vi "PicoScope2000aExampleRapidBlock.vi"() -> ()   [LabVIEW 2009]
panel:
  in  "Channel A Settings":T1 {"Range" items=["20 mV", "50 mV", "100 mV", "200 mV", "500 mV", "1 V", "2 V", "5 V", "10 V", "20 V"]; "Coupling" items=["AC", "DC"]}
  out "Properties Panel":T2 {"Max Total Capture Time Available (sec)" format="%.3p"; "Sample Frequency" format="%.3p"; "Sample Internal" format="%.3p"; "Max Samples Available" format="%.3p"; "Total Capture Time (sec)" format="%.3p"}
  in  "Down Sample Ratio":u32 min=1 step=1
  in  "Down-Sample Mode":i32(ring) items=["None", "Aggregate", "Decimate", "Average"]
  in  "Trigger Settings":T3 {"Trigger Direction" items=["Rising", "Falling"]}
  in  "Rapid Block Acquisition Settings":T4
  out "Capture Complete":bool
  in  "Run":bool
  out "Channel A":T5(graph)
  in  "Capture Index":u32
  in  "stop":bool
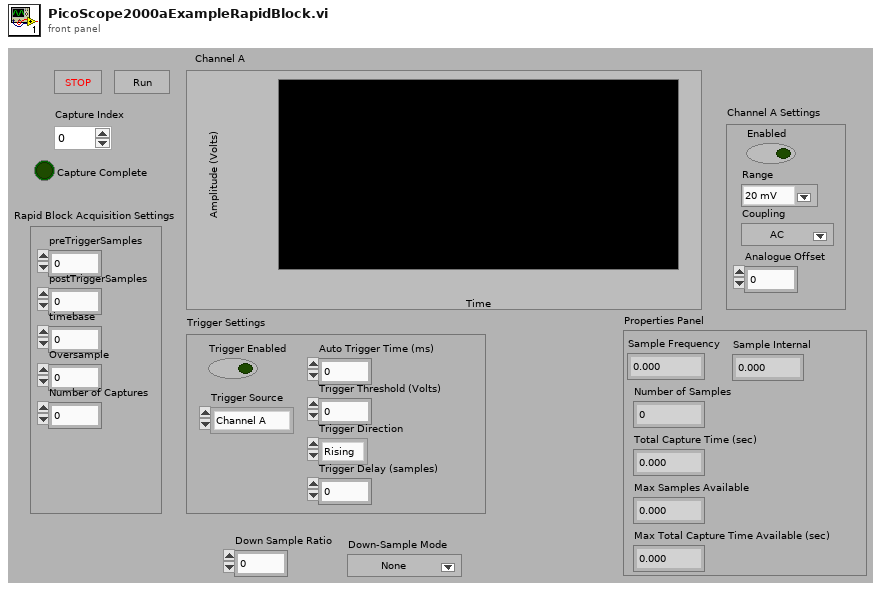
[diagram p1: front panel]
types:
  T1 = cluster{"Enabled":bool, "Coupling":i16, "Range":u16, "Analogue Offset":sgl}
  T2 = cluster{"Sample Frequency":sgl, "Sample Internal":sgl, "Max Samples Available":i32, "Number of Samples":u32, "Total Capture Time (sec) ":sgl, "Max Total Capture Time Available (sec)":sgl}
  T3 = cluster{"Trigger Enabled":bool, "Trigger Source":enum16{"Channel A", "Channel B", "Channel C", "Channel D", "Ext."}, "Trigger Threshold (Volts)":dbl, "Trigger Direction":u16, "Trigger Delay (samples)":u32, "Auto Trigger Time (ms)":i16}
  T4 = cluster{"preTriggerSamples":u32, "postTriggerSamples":u32, "timebase":u32, "Oversample":i16, "Number of Captures":u32}
  T5 = cluster{i32, "Sample Internal":sgl, "Data (Volts)":dbl[]}
  T6 = cluster{"Driver Version":string, "USB Version":string, "Hardware":string, "Variant":string, "Batch and Serial":string, "Cal Date":string, "Kernel Version":string, "Digital HW Version":string, "Analogue HW Version":string, "Firmware 1":string, "Firmware 2":string, "MSO":bool, "Number of Channels":i16}
  T7 = cluster{"preTriggerSamples":u32, "postTriggerSamples":u32, "timebase":u32, "Down-Sample Mode":i32, "Down Sample Ratio":u32, i16}
  T8 = cluster{i32, "Sample Internal":sgl, "Data":dbl[]}
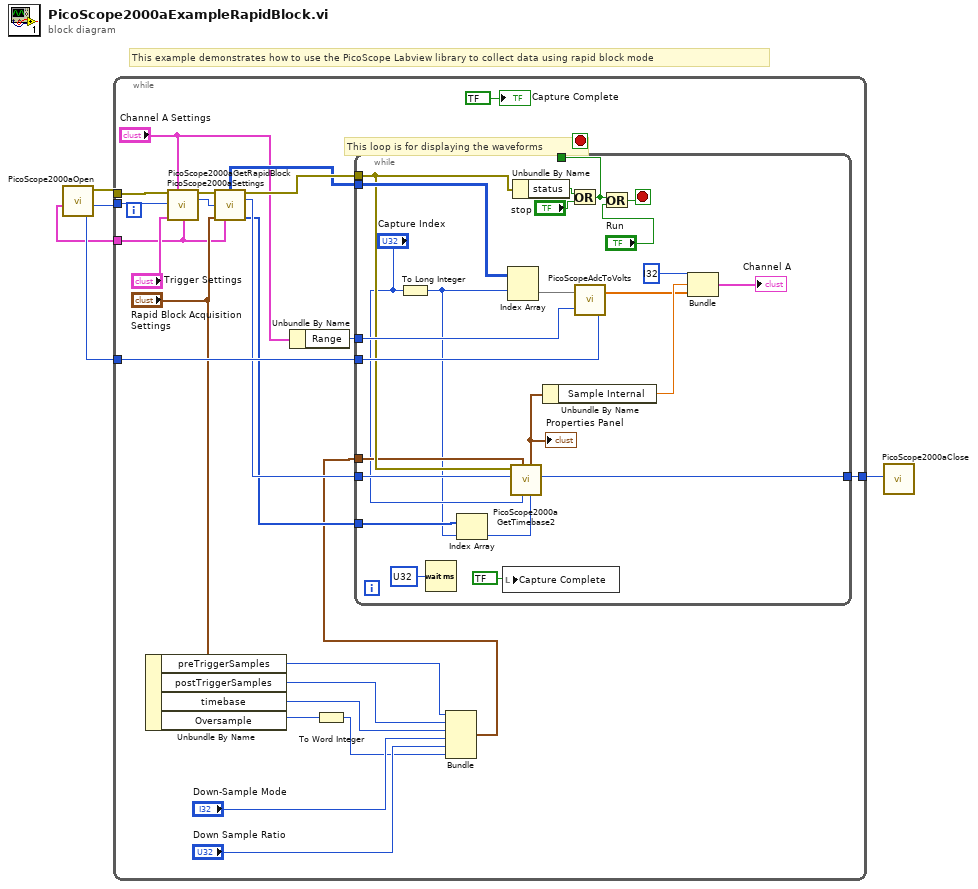
[diagram p0: block diagram]
diagram:
  # "This example demonstrates how to use the PicoScope Labview library to collect data using rapid block mode"
  n1 = call "PicoScope2000aOpen.vi"() -> ("Max Adc value"=w3:i16, "handle"=w4:i16, "error out"=w5:errorcluster, "Device Info"=w1:T6)  [unwired: 4 in]
  n2 = while {
    tunnel: w4 -> [w27]
    tunnel: w5 -> [w28]
    tunnel: w3 -> [w22]
    tunnel: [w18] -> w2
    tunnel: w1 -> [w7]
    stop <- w30 stop-if-true
    # "This loop is for displaying the waveforms"
    n3 = Unbundle By Name("Rapid Block Acquisition Settings") -> ("preTriggerSamples"=w15:u32, "postTriggerSamples"=w14:u32, "timebase"=w13:u32, "Oversample"=w12:i16)
    n4 = call "PicoScope2000aSettings.vi"("error in"=w28, "Channel A Settings"="Channel A Settings", "handle in"=w27, "Trigger Settings"="Trigger Settings", "Device Info"=w7) -> ("error out"=w23:errorcluster, "handle out"=w24:i16)  [unwired: 8 in, 1 out]
    n5 = call "PicoScope2000aGetRapidBlock.vi"("error in"=w23, "handle in"=w24, "Rapid Block Acquisition Settings"="Rapid Block Acquisition Settings", "Device Info"=w7) -> ("Channel A Buffer"=w25:i16[][], "error out"=w26:errorcluster, "handle out"=w19:i16, "noOfSamples Array"=w17:u32[])  [unwired: 5 in, 3 out]
    n6 = Unbundle By Name("Channel A Settings") -> ("Range"=w21:u16)
    n7 = To Word Integer(number=w12) -> (16bit integer=w8:i16)
    n8 = Bundle("preTriggerSamples"=w15, "postTriggerSamples"=w14, "timebase"=w13, "Down-Sample Mode"="Down-Sample Mode", "Down Sample Ratio"="Down Sample Ratio", w8) -> (w16:T7)  [unwired: 1 in]
    n9 = while {
      tunnel: [w53] -> w30
      tunnel: w25 -> [w47]
      tunnel: w26 -> [w43]
      tunnel: w22 -> [w46]
      tunnel: w21 -> [w44]
      tunnel: w16 -> [w38]
      tunnel: w19 -> [w42]
      tunnel: [w41] -> w18
      tunnel: w17 -> [w40]
      stop <- w52 stop-if-true
      n10 = To Long Integer(number="Capture Index") -> (32bit integer=w36:i32)
      n11 = Wait (ms)(milliseconds to wait=u32 ?) -> ()  [unwired: 1 out]
      n12 = Index Array(array=w40, index=w36) -> (element=w39:u32)
      n13 = local write "Capture Complete"(bool ? ("Capture Complete")) -> ()
      n14 = Index Array(array=w47, index (row)=w36) -> (element=w45:i16[])  [unwired: 1 in]
      n15 = call "PicoScope2000aGetTimebase2.vi"("Number of Samples"=w39, "Memory Segment"="Capture Index", "Acquisition Settings"=w38, "handle in"=w42, "error in (no error)"=w43) -> ("handle out"=w41:i16, "Properties Panel"=w33:T2)  [unwired: 4 in, 1 out]
      "Properties Panel" <- w33
      n16 = Unbundle By Name(w43) -> ("status"=w48:bool)
      n17 = Unbundle By Name(w33) -> ("Sample Internal"=w34:sgl)
      n18 = Or(x=w48, y="stop") -> (x .or. y?=w53:bool)
      n19 = call "PicoScopeAdcToVolts.vi"("Max_adc"=w46, "Range Index"=w44, "Data"=w45) -> ("Data"=w32:dbl[])
      n20 = Or(x=w53, y="Run") -> (x .or. y?=w52:bool)
      n21 = Bundle(i32 ?, "Sample Internal"=w34, "Data"=w32) -> (→"Channel A":T8)  [unwired: 1 in]
    }
    "Capture Complete" <- bool ? ("Capture Complete")
  }
  n22 = call "PicoScope2000aClose.vi"("handle"=w2) -> ()
